vi "interfazlabviewcarrito.vi"() -> ()   [LabVIEW 2019]
uses:
  <vilib>/regexp/Match Regular Expression.xnode
  <vilib>/Utility/file.llb/Write Delimited Spreadsheet (DBL).vi
  <vilib>/Instr/_visa.llb/VISA Configure Serial Port (Instr).vi
panel:
  out "Referencia":dbl
  out "Salida":dbl
  out "Esfuerzo de control":dbl
  out "Tiempo":dbl
  out "Datos a tomar del serial":string
  out "Datos seriales del arduino":string
  out "Waveform Chart":dbl[][](graph)
  out "error out":errorcluster
  in  "stop":bool
  in  "REFERENCIA":dbl
  in  "VISA resource name":refnum<visa-resource-name>
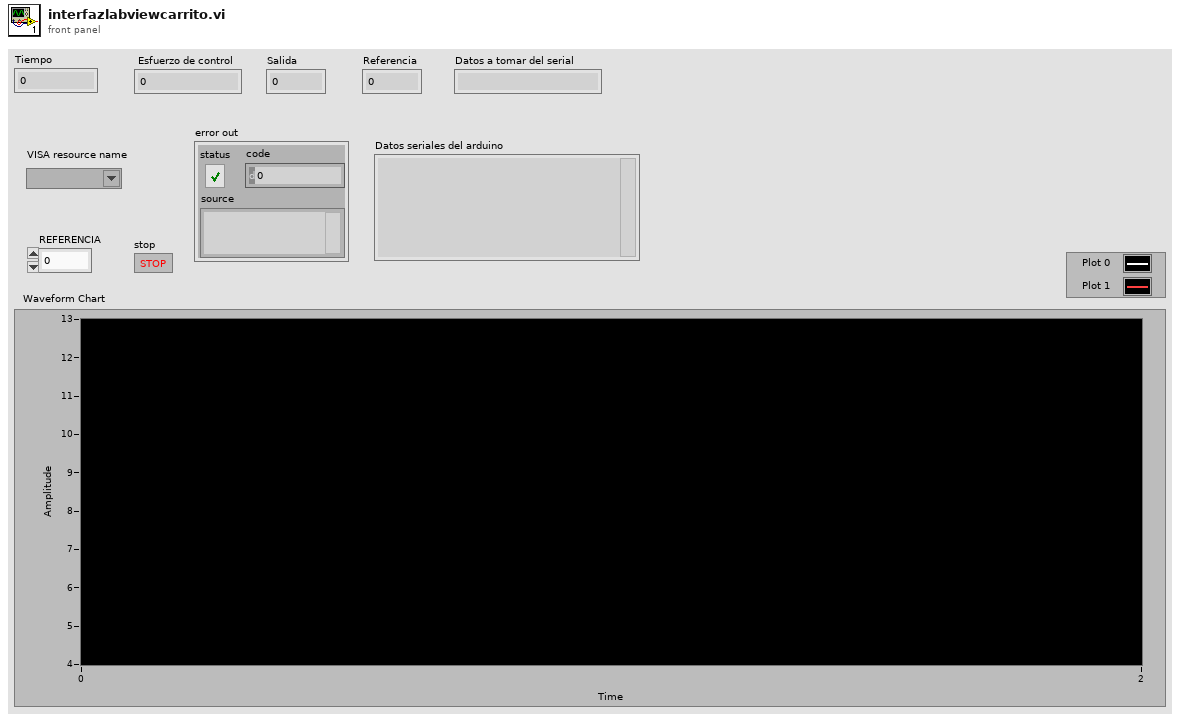
[diagram p1: front panel]
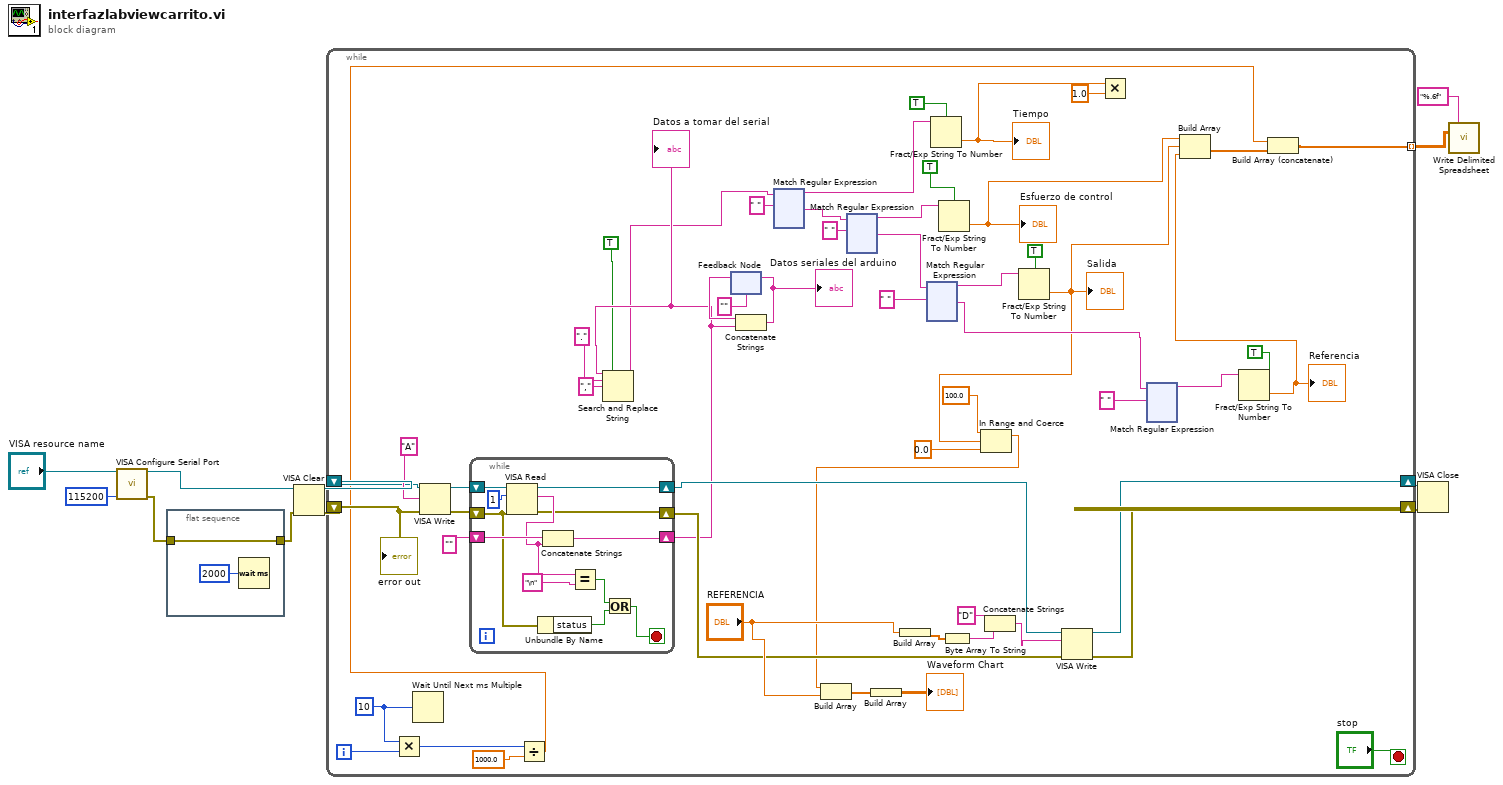
[diagram p0: block diagram]
diagram:
  n1 = call-poly "VISA Configure Serial Port"("VISA resource name"="VISA resource name", "baud rate (9600)"=u32 115200) -> ("VISA resource name out"=w7:refnum<visa-resource-name>, "error out"=w10:errorcluster)  [unwired: 12 in]
  n2 = flat-sequence {
    tunnel: w10 -> [w12]
    tunnel: [w12] -> w5
    frame #0 {
      n3 = Wait (ms)(milliseconds to wait=u32 2000) -> ()  [unwired: 1 out]
    }
  }
  n4 = VISA Clear(VISA resource name=w7, error in (no error)=w5) -> (VISA resource name out=w6:refnum<visa-resource-name>, error out=w4:errorcluster)
  n5 = while {
    shift-right: [w64] -> w9
    shift-left: w6 -> [w59]
    shift-right: [w63] -> w8
    shift-left: w4 -> [w58]
    tunnel: [w16] -> w2 mode=indexing
    i -> [w17]
    stop <- "stop" stop-if-true
    w20 = u32 10 ("millisecond multiple")
    n6 = Multiply(x=w20, y=w17) -> (x*y=w18:u32)
    n7 = Wait Until Next ms Multiple(millisecond multiple=w20) -> ()  [unwired: 1 out]
    n8 = VISA Write(VISA resource name=w59, write buffer="A", error in (no error)=w58) -> (VISA resource name out=w52:refnum<visa-resource-name>, error out=w51:errorcluster)  [unwired: 1 out]
    n9 = while {
      shift-right: [w539] -> w49
      shift-left: w52 -> [w549]
      shift-right: [w538] -> w50
      shift-left: w51 -> [w543]
      shift-right: [w547] -> w44
      shift-left: "" -> [w546]
      stop <- w540 stop-if-true
      n10 = VISA Read(VISA resource name=w549, byte count=u32 1, error in (no error)=w543) -> (VISA resource name out=w539:refnum<visa-resource-name>, read buffer=w545:string, error out=w538:errorcluster)  [unwired: 1 out]
      n11 = Unbundle By Name(w543) -> ("status"=w541:bool)
      n12 = Concatenate Strings(w546, w545) -> (w547:string)
      n13 = Equal?(x=w545, y="\n") -> (x = y?=w542:bool)
      n14 = Or(x=w542, y=w541) -> (x .or. y?=w540:bool)
    }
    "Datos a tomar del serial" <- w44
    n15 = Divide(x=w18, y=1000.0) -> (x/y=w14:dbl)
    n16 = Search and Replace String(replace all?=TRUE ("replace all? (F)"), input string=w44, search string="." ("substring (\"\")"), replace string="," ("replace string (\"\")")) -> (result string=w40:string)  [unwired: 4 in, 3 out]
    n17 = feedback #1("") -> (w55:string)
    n18 = Concatenate Strings(w55, w44) -> (w56:string)
    "Datos seriales del arduino" <- w56
    n19 = feedback-in #1(w56) -> ()
    n20 = xnode "Match Regular Expression"("input string"=w40, "regular expression"=" ") -> ("before match"=w39:string, "after match"=w46:string)  [unwired: 4 in, 3 out]
    n21 = xnode "Match Regular Expression"("input string"=w46, "regular expression"=" ") -> ("before match"=w37:string, "after match"=w34:string)  [unwired: 4 in, 3 out]
    n22 = Build Array("REFERENCIA") -> (w68:dbl[])
    n23 = xnode "Match Regular Expression"("input string"=w34, "regular expression"=" ") -> ("before match"=w36:string, "after match"=w29:string)  [unwired: 4 in, 3 out]
    n24 = Fract/Exp String To Number(use system decimal point (T)=TRUE, string=w39) -> (number=w27:dbl)  [unwired: 2 in, 1 out]
    "Tiempo" <- w27
    n25 = Fract/Exp String To Number(use system decimal point (T)=TRUE, string=w37) -> (number=w28:dbl)  [unwired: 2 in, 1 out]
    "Esfuerzo de control" <- w28
    n26 = Byte Array To String(unsigned byte array=w68) -> (string=w67:string)
    n27 = Concatenate Strings("D" ("string"), w67) -> (w65:string)
    n28 = Fract/Exp String To Number(use system decimal point (T)=TRUE, string=w36) -> (number=w22:dbl)  [unwired: 2 in, 1 out]
    "Salida" <- w22
    n29 = In Range and Coerce(upper limit=100.0, x=w22, lower limit=0.0) -> (coerced(x)=w21:dbl)  [unwired: 1 out]
    n30 = Build Array(w21, "REFERENCIA") -> (w60:dbl[])
    n31 = Build Array(w60) -> (→"Waveform Chart":dbl[][])
    n32 = VISA Write(VISA resource name=w49, write buffer=w65, error in (no error)=w50) -> (VISA resource name out=w64:refnum<visa-resource-name>, error out=w63:errorcluster)  [unwired: 1 out]
    n33 = Multiply(x=w27, y=1.0) -> ()  [unwired: 1 out]
    n34 = xnode "Match Regular Expression"("input string"=w29, "regular expression"=" ") -> ("before match"=w32:string)  [unwired: 4 in, 4 out]
    n35 = Fract/Exp String To Number(use system decimal point (T)=TRUE, string=w32) -> (number=w25:dbl)  [unwired: 2 in, 1 out]
    "Referencia" <- w25
    n36 = Build Array(w28, w22, w25) -> (w15:dbl[])
    n37 = Build Array (concatenate)(w14, w15) -> (w16:dbl[])
    "error out" <- w58
  }
  n38 = VISA Close(VISA resource name=w9, error in (no error)=w8) -> ()  [unwired: 1 out]
  n39 = call-poly <vilib>:"Write Delimited Spreadsheet.vi"("format (%.3f)"="%.6f", "2D data"=w2) -> ()  [unwired: 12 in, 2 out]
